vi "DriveFwdAuto.vi"(8 "error in":errorcluster, 9 "Timeout":dbl, 10 "MaxSpeed":dbl, 11 "Distance":dbl) -> (0 "error out":errorcluster, 3 "Done":bool)   [LabVIEW 2020]
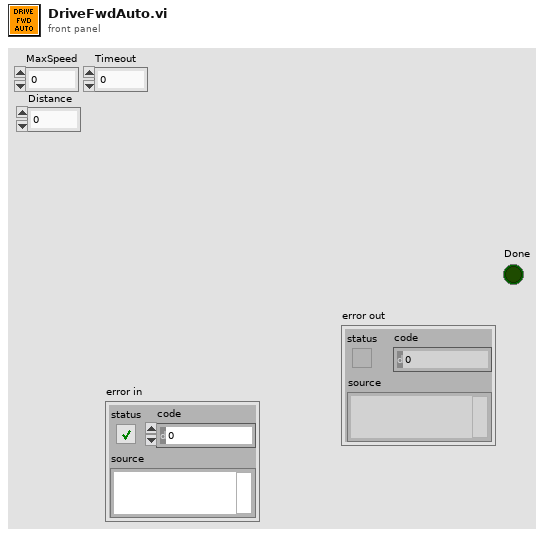
[diagram p1: front panel]
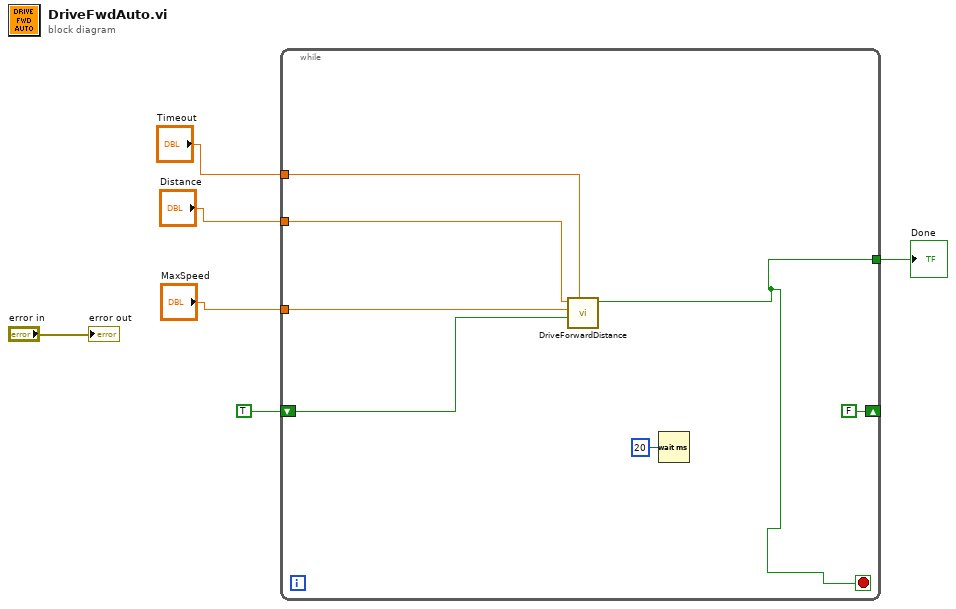
[diagram p0: block diagram]
diagram:
  n1 = while {
    tunnel: [w8] -> w5
    tunnel: "MaxSpeed" -> [w13]
    tunnel: "Distance" -> [w12]
    tunnel: "Timeout" -> [w11]
    shift-right: [FALSE] -> _
    shift-left: TRUE -> [w10]
    stop <- w8 stop-if-true
    n2 = call "DriveForwardDistance.vi"("Timeout"=w11, "Initation?"=w10, "MaxSpeed"=w13, "Distance"=w12) -> ("Finished"=w8:bool)  [unwired: 5 in, 2 out]
    n3 = Wait (ms)(milliseconds to wait=u32 20) -> ()  [unwired: 1 out]
  }
  "Done" <- w5
  "error out" <- "error in"
